vi "AIT 664 - Read FIFOs.vi"(0 "RT Data in":T2 {"End System Handle" format="%x"; "Label Transfer Config"."Block Data Refs"."Data Reference" format="%.0x"; "Status Config"."Hardware Out Dur Reference" format="%.0x"; "Status Config"."Hardware In Dur Reference" format="%.0x"; "Status Config"."Hardware Out Count Reference" format="%.0x"; "Status Config"."Hardware In Count Reference" format="%.0x"; "Status Config"."Error Data Reference" format="%.0x"; "Hardware Output Tx Channels"."Message Settings"."Transmit Channel Data Reference" format="%.0x"; "Hardware Output Tx Channels"."Message Settings"."Queue Transmit Channel" format="%.0x"; "Hardware Output Tx Channels"."Message Settings"."Driver Data"."Num Bits" min=1 max=32; "Hardware Output Tx Channels"."Message Settings"."Block Data Refs"."Data Reference" format="%.0x"; "Hardware Output Tx Channels"."Rx Com Udp Port"."Handle" format="%08x"; "Hardware Output Tx Channels"."Tx Com Udp Port"."Handle" format="%08x"; "Hardware Input Rx Channels"."Message Settings"."Transmit Channel Data Reference" format="%.0x"; "Hardware Input Rx Channels"."Message Settings"."Queue Transmit Channel" format="%.0x"; "Hardware Input Rx Channels"."Message Settings"."Driver Data"."Num Bits" min=1 max=32; "Hardware Input Rx Channels"."Message Settings"."Block Data Refs"."Data Reference" format="%.0x"; "Hardware Input Rx Channels"."Rx Com Udp Port"."Handle" format="%08x"; "Hardware Input Rx Channels"."Tx Com Udp Port"."Handle" format="%08x"}, 1 "Mode":T1, 5 "Channel Index":i32, 11 "error in (no error)":errorcluster) -> (4 "RT Data out":T2 {"End System Handle" format="%x"; "Label Transfer Config"."Block Data Refs"."Data Reference" format="%.0x"; "Status Config"."Hardware Out Dur Reference" format="%.0x"; "Status Config"."Hardware In Dur Reference" format="%.0x"; "Status Config"."Hardware Out Count Reference" format="%.0x"; "Status Config"."Hardware In Count Reference" format="%.0x"; "Status Config"."Error Data Reference" format="%.0x"; "Hardware Output Tx Channels"."Message Settings"."Transmit Channel Data Reference" format="%.0x"; "Hardware Output Tx Channels"."Message Settings"."Queue Transmit Channel" format="%.0x"; "Hardware Output Tx Channels"."Message Settings"."Driver Data"."Num Bits" min=1 max=32; "Hardware Output Tx Channels"."Message Settings"."Block Data Refs"."Data Reference" format="%.0x"; "Hardware Output Tx Channels"."Rx Com Udp Port"."Handle" format="%08x"; "Hardware Output Tx Channels"."Tx Com Udp Port"."Handle" format="%08x"; "Hardware Input Rx Channels"."Message Settings"."Transmit Channel Data Reference" format="%.0x"; "Hardware Input Rx Channels"."Message Settings"."Queue Transmit Channel" format="%.0x"; "Hardware Input Rx Channels"."Message Settings"."Driver Data"."Num Bits" min=1 max=32; "Hardware Input Rx Channels"."Message Settings"."Block Data Refs"."Data Reference" format="%.0x"; "Hardware Input Rx Channels"."Rx Com Udp Port"."Handle" format="%08x"; "Hardware Input Rx Channels"."Tx Com Udp Port"."Handle" format="%08x"}, 15 "error out":errorcluster)   [LabVIEW 2013, in "AIT 664 Custom Device.lvlib"]
doc: "Move data from the FIFOs to the buffers to then be moved to veristand or the hardware.\n\nInline Read - Move data from the Hardware In FIFO to the Hardware In Buffer and onto Veristand\nAsync HWOut - Move data from Hardware Out FIFO to the Hardware Out Buffer and onto the device write"
uses:
  AIT 664 Custom Device.lvlib
  RT Controls/AIT 664  - RT Data.ctl
  RT Controls/AIT 664 - RT Hardware Channel.ctl
  RT Controls/AIT 664 - RT Message Settings.ctl
  <vilib>/NI Veristand/Custom Device API/Block Data Reference.ctl
  <vilib>/NI Veristand/Custom Device API/Data Reference.ctl
  RT Controls/AIT 664 - Driver Data.ctl
  Controls and Global/Start Bit.ctl
  Controls and Global/Number of Bits.ctl
  <vilib>/NI Veristand/Custom Device API/Custom Device Item Ref.ctl
  <userlib>/ARINC 664/AIT 664 Controls/General/Message Port.ctl
  <userlib>/ARINC 664/AIT 664 Controls/General/Direction.ctl
  <userlib>/ARINC 664/AIT 664 Controls/General/Message Port Type.ctl
  System Explorer/Controls/664 - Sampling Type.ctl
  RT Controls/Status Channels Config.ctl
  RT Controls/FIFO.ctl
  RT Controls/Label Transfer Config.ctl
  RT Controls/ReadWrite Selector.ctl
  <vilib>/NI Veristand/Custom Device API/Custom Device API.lvlib
  <userlib>/ARINC 664/AIT 664 API.lvlib
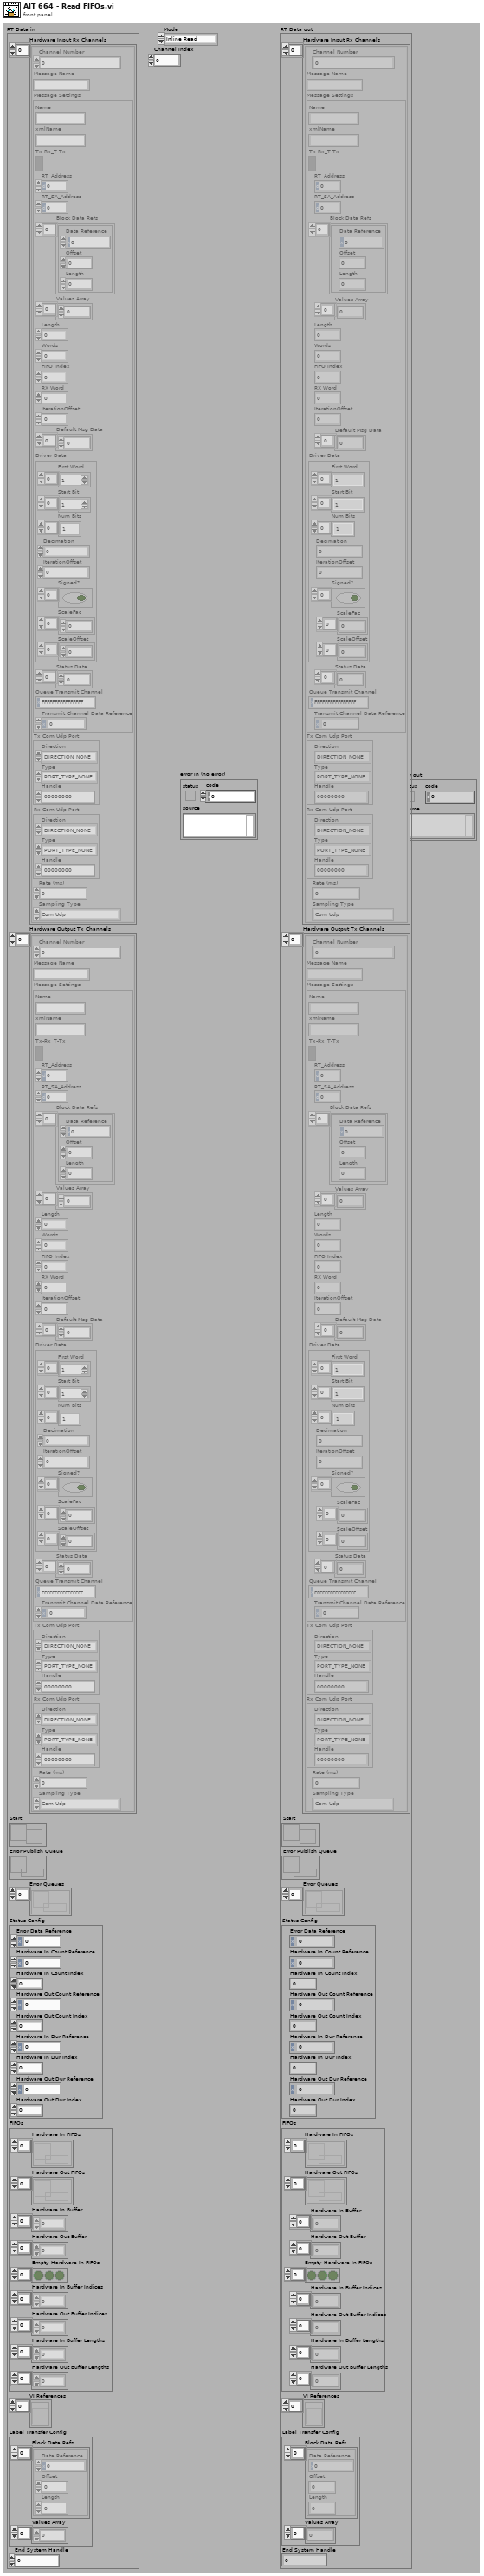
[diagram p1: front panel]
types:
  T1 = typedef "AIT 664 Custom Device.lvlib/ReadWrite Selector.ctl" = enum16{"Inline Read", "Inline Write", "Async HWIn", "Async HWOut"}
  T2 = typedef "AIT 664 Custom Device.lvlib/AIT 664  - RT Data.ctl" = cluster{"Hardware Input Rx Channels":T3[], "Hardware Output Tx Channels":T3[], "Start":refnum<notifier>, "Error Publish Queue":refnum<queue>, "Error Queues":refnum<queue>[], "Status Config":T15, "FIFOs":T16, "VI References":refnum<vi>[], "Label Transfer Config":T17, "End System Handle ":u64}
  T3 = typedef "AIT 664 Custom Device.lvlib/AIT 664 - RT Hardware Channel.ctl" = cluster{"Channel Number":u16, "Message Name":string, "Message Settings":T4, "Tx Com Udp Port":T11, "Rx Com Udp Port":T11, "Rate (ms)":u32, "Sampling Type":T14}
  T4 = typedef "AIT 664 Custom Device.lvlib/AIT 664 - RT Message Settings.ctl" = cluster{"Name":string, "xmlName":string, "Tx-Rx_T-Tx":bool, "RT_Address":u8, "RT_SA_Address":u8, "Block Data Refs":T5[], "Values Array":dbl[], "Length":i32, "Words":i32, "FIFO Index":i32, "RX Word":u32, "IterationOffset":i32, "Default Msg Data":u8[], "Driver Data":T7, "Status Data":u32[], "Queue Transmit Channel":T10, "Transmit Channel Data Reference":T6}
  T5 = typedef "Custom Device API.lvlib/Block Data Reference.ctl" = cluster{"Data Reference":T6, "Offset":i32, "Length":i32}
  T6 = typedef "Custom Device API.lvlib/Data Reference.ctl" = i32
  T7 = typedef "AIT 664 Custom Device.lvlib/AIT 664 - Driver Data.ctl" = cluster{"First Word":T8[], "Start Bit":T8[], "Num Bits":T9[], "Decimation":i32, "IterationOffset":i32, "Signed?":bool[], "ScaleFac":dbl[], "ScaleOffset":dbl[]}
  T8 = typedef "AIT 664 Custom Device.lvlib/Start Bit.ctl" = i32
  T9 = typedef "AIT 664 Custom Device.lvlib/Number of Bits.ctl" = i32
  T10 = typedef "Custom Device API.lvlib/Custom Device Item Ref.ctl" = u64
  T11 = typedef "AIT 664 API.lvlib/Message Port.ctl" = cluster{"Direction":T12, "Type":T13, "Handle":u64}
  T12 = typedef "AIT 664 API.lvlib/Direction.ctl" = enum16{"DIRECTION_NONE", "DIRECTION_TX", "DIRECTION_RX"}
  T13 = typedef "AIT 664 API.lvlib/Message Port Type.ctl" = enum16{"PORT_TYPE_NONE", "COM_UDP", "SAP_UDP", "SAP_IP", "SAP_MAC", "COTS_MAC", "COTS_MAC_RAW"}
  T14 = typedef "AIT 664 Custom Device.lvlib/664 - Sampling Type.ctl" = enum16{"Com Udp", "Com Udp Queuing", "Sap Udp", "Sap Ip", "Sap Mac", "Unknown"}
  T15 = typedef "AIT 664 Custom Device.lvlib/Status Channels Config.ctl" = cluster{"Error Data Reference":T6, "Hardware In Count Reference":T6, "Hardware In Count Index":i32, "Hardware Out Count Reference":T6, "Hardware Out Count Index":i32, "Hardware In Dur Reference":T6, "Hardware In Dur Index":i32, "Hardware Out Dur Reference":T6, "Hardware Out Dur Index":i32}
  T16 = typedef "AIT 664 Custom Device.lvlib/FIFO.ctl" = cluster{"Hardware In FIFOs":refnum<k33>[], "Hardware Out FIFOs":refnum<k33>[], "Hardware In Buffer":dbl[], "Hardware Out Buffer":dbl[], "Empty Hardware In FIFOs":bool[], "Hardware In Buffer Indices":i32[], "Hardware Out Buffer Indices":i32[], "Hardware In Buffer Lengths":i32[], "Hardware Out Buffer Lengths":i32[]}
  T17 = typedef "AIT 664 Custom Device.lvlib/Label Transfer Config.ctl" = cluster{"Block Data Refs":T5[], "Values Array":dbl[]}
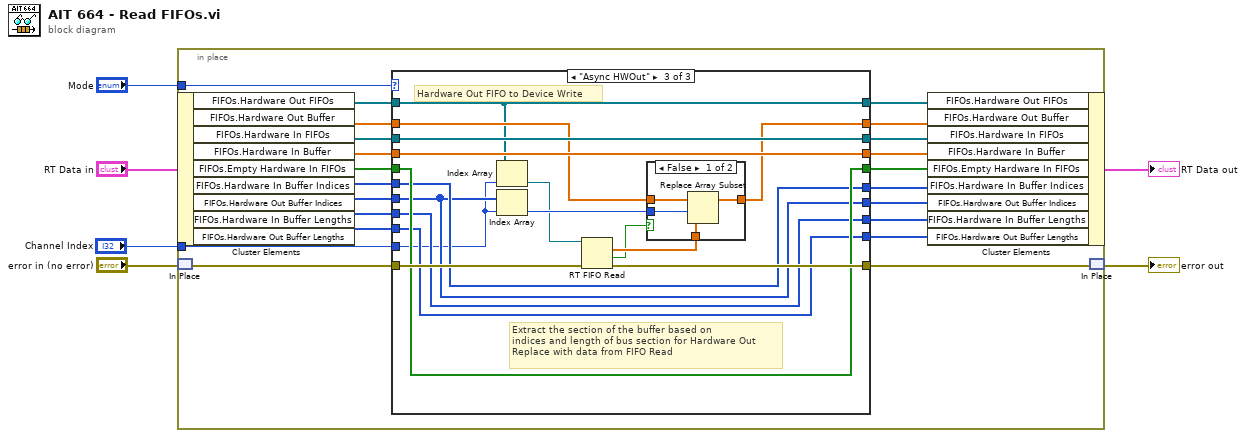
[diagram p0: block diagram]
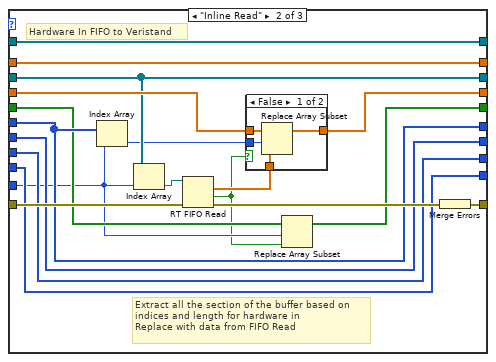
[diagram p3: hidden frame]
diagram:
  n1 = in-place {
    in-place-border: "Mode" -> [w21]
    in-place-border: "Channel Index" -> [w13]
    n2 = in-place-cluster #1("RT Data in") -> ("FIFOs.Hardware Out FIFOs"=w19:refnum<k33>[], "FIFOs.Hardware Out Buffer"=w18:dbl[], "FIFOs.Hardware In FIFOs"=w28:refnum<k33>[], "FIFOs.Hardware In Buffer"=w27:dbl[], "FIFOs.Empty Hardware In FIFOs"=w20:bool[], "FIFOs.Hardware In Buffer Indices"=w12:i32[], "FIFOs.Hardware Out Buffer Indices"=w15:i32[], "FIFOs.Hardware In Buffer Lengths"=w9:i32[], "FIFOs.Hardware Out Buffer Lengths"=w14:i32[])
    n3 = in-place-match #2("error in (no error)") -> (w23:errorcluster)
    n4 = case shown="\"Async HWOut\"" w21 {
      tunnel: w28 -> [w37 w46 w76]
      tunnel: w27 -> [w38 w50 w77]
      tunnel: [w38 w48 w77] -> w26
      tunnel: [w37 w46 w76] -> w25
      tunnel: [w36 w39 w75] -> w24
      tunnel: w23 -> [w35 w57 w79]
      tunnel: [w35 w49 w78] -> w22
      tunnel: w20 -> [w36 w42 w75]
      tunnel: w19 -> [w33 w54 w66]
      tunnel: w18 -> [w34 w55 w74]
      tunnel: [w33 w54 w66] -> w17
      tunnel: [w34 w55 w71] -> w16
      tunnel: w15 -> [w31 w53 w69]
      tunnel: w14 -> [w29 w52 w67]
      tunnel: w13 -> [_ w41 w65]
      tunnel: [w32 w44 w70] -> w11
      tunnel: w12 -> [w32 w44 w70]
      tunnel: [w31 w53 w69] -> w10
      tunnel: [w30 w51 w68] -> w8
      tunnel: w9 -> [w30 w51 w68]
      tunnel: [w29 w52 w67] -> w7
      frame Default {
      }
      frame "Inline Read" {
        # "Hardware In FIFO to Veristand"
        # "Extract all the section of the buffer based on \nindices and length for hardware in\nReplace with data from FIFO Read"
        n5 = Index Array(array=w44, index=w41) -> (element=w43:i32)
        n6 = Index Array(array=w46, index=w41) -> (element=w45:refnum<k33>)
        n7 = RT FIFO Read(0:w45, 3:w57) -> (9:w47:dbl[], 10:w40:bool, 11:w56:errorcluster)  [unwired: 2 in, 2 out]
        n8 = case shown="False" w40 {
          tunnel: w47 -> [w61 _]
          tunnel: w43 -> [w60 _]
          tunnel: w50 -> [w59 w62]
          tunnel: [w58 w62] -> w48
          frame False {
            n9 = Replace Array Subset(array=w59, new element=w61, index=w60) -> (w58:dbl[])
          }
          frame True {
          }
        }
        n10 = Replace Array Subset(array=w42, new element=w40, index=w41) -> (w39:bool[])
        n11 = Merge Errors(w56) -> (w49:errorcluster)
      }
      frame "Async HWOut" {
        # "Hardware Out FIFO to Device Write"
        # "Extract the section of the buffer based on \nindices and length of bus section for Hardware Out\nReplace with data from FIFO Read"
        n12 = Index Array(array=w66, index=w65) -> (element=w64:refnum<k33>)
        n13 = Index Array(array=w69, index=w65) -> (element=w73:i32)
        n14 = RT FIFO Read(0:w64, 3:w79) -> (9:w72:dbl[], 10:w63:bool, 11:w78:errorcluster)  [unwired: 2 in, 2 out]
        n15 = case shown="False" w63 {
          tunnel: w74 -> [w83 w84]
          tunnel: w73 -> [w82 _]
          tunnel: w72 -> [w81 _]
          tunnel: [w80 w84] -> w71
          frame False {
            n16 = Replace Array Subset(array=w83, new element=w81, index=w82) -> (w80:dbl[])
          }
          frame True {
          }
        }
      }
    }
    n17 = in-place-cluster #1("FIFOs.Hardware Out FIFOs"=w17, "FIFOs.Hardware Out Buffer"=w16, "FIFOs.Hardware In FIFOs"=w25, "FIFOs.Hardware In Buffer"=w26, "FIFOs.Empty Hardware In FIFOs"=w24, "FIFOs.Hardware In Buffer Indices"=w11, "FIFOs.Hardware Out Buffer Indices"=w10, "FIFOs.Hardware In Buffer Lengths"=w8, "FIFOs.Hardware Out Buffer Lengths"=w7) -> (→"RT Data out":T2)
    n18 = in-place-match #2(w22) -> (→"error out":errorcluster)
  }
